vi "MCListbox Edit Reference.vi"(6 "EditPos In":T1, 7 "Get/Set":enum16{"Get", "Set"}(ring)=enum."Set", 8 "Error In":errorcluster, 9 "Ctl Ref String":string, 10 "MCListBox In":refnum<vi>, 11 "MCListBox Related Ref In":refnum<vi>[](array[refnum])) -> (0 "Error Out":errorcluster, 2 "MCListBox Out":refnum<vi>, 3 "MCListBox Related Ref Out":refnum<vi>[](array[refnum]), 4 "EditPos Out":T1)   [LabVIEW 2013]
uses:
  <vilib>/Utility/miscctls.llb/LVRowAndColumnTypeDef.ctl
panel:
  out "Array":string[](array[string])
  out "Class Name":string
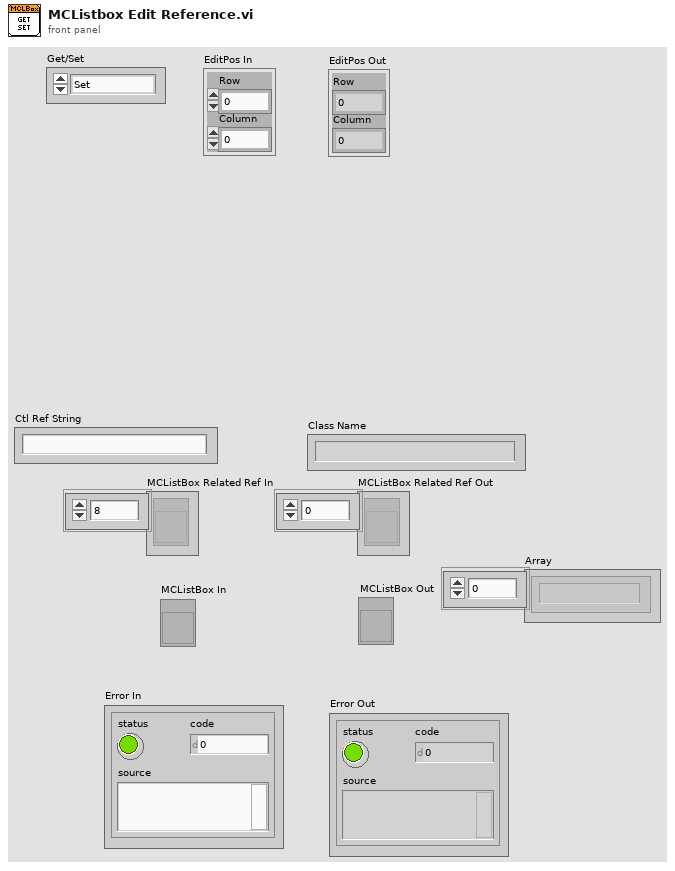
[diagram p1: front panel]
types:
  T1 = typedef "LVRowAndColumnTypeDef.ctl" = cluster{"Row":i32, "Column":i32}
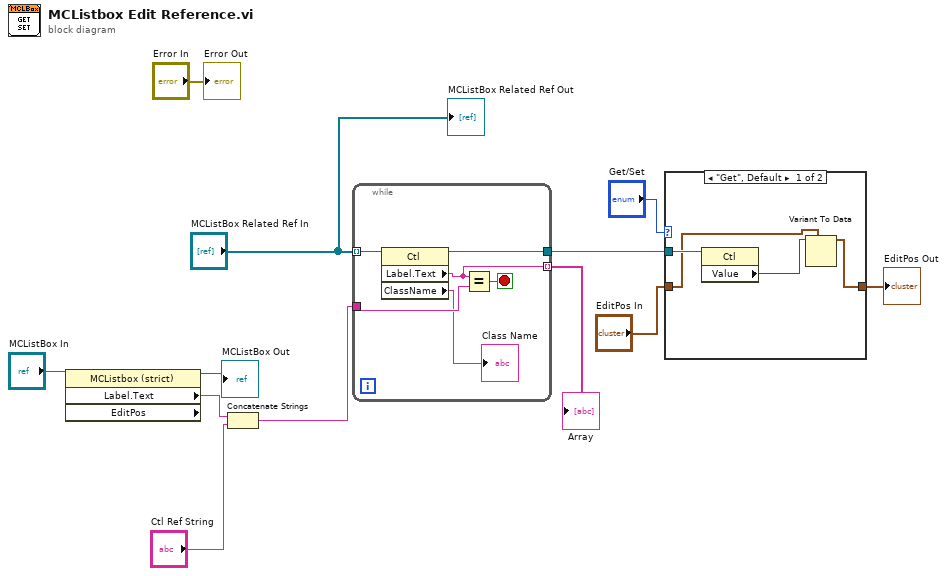
[diagram p0: block diagram]
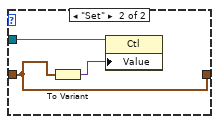
[diagram p2: hidden frame]
diagram:
  n1 = property on="Property Node" class="MCListbox (strict)" props=["Label", "Text", "EditPos"](reference="MCListBox In") -> (reference out=→"MCListBox Out":refnum<vi>, "Label.Text"=w8:string)  [unwired: 1 in, 2 out]
  n2 = Concatenate Strings(w8, "Ctl Ref String") -> (w6:string)
  n3 = while {
    tunnel: "MCListBox Related Ref In" -> [w18] mode=indexing
    tunnel: w6 -> [w17]
    tunnel: [w15] -> w5
    tunnel: [w13] -> w4 mode=indexing
    stop <- w16 stop-if-true
    n4 = property on="Property Node" class="Ctl"(reference=w18) -> (reference out=w15:refnum<vi>, "Label.Text"=w13:string, "ClassName"=→"Class Name":string)  [unwired: 1 in, 1 out]
    n5 = Equal?(x=w13, y=w17) -> (x = y?=w16:bool)
  }
  "Array" <- w4
  n6 = case shown="\"Get\", Default" "Get/Set" {
    tunnel: w5 -> [w22 w25]
    tunnel: "EditPos In" -> [w20 w24]
    tunnel: [w19 w24] -> w11
    frame "Get", Default {
      n7 = property on="Property Node" class="Ctl"(reference=w22) -> ("Value"=w21:variant)  [unwired: 1 in, 2 out]
      n8 = Variant To Data(type=w20, Variant=w21) -> (data=w19:T1)  [unwired: 1 in, 1 out]
    }
    frame "Set" {
      n9 = To Variant(anything=w24) -> (Variant=w23:variant)
      n10 = property on="Property Node" class="Ctl"(reference=w25, "Value"=w23) -> ()  [unwired: 1 in, 2 out]
    }
  }
  "EditPos Out" <- w11
  "Error Out" <- "Error In"
  "MCListBox Related Ref Out" <- "MCListBox Related Ref In"
